vi "GetText.vi"(8 "error in":errorcluster, 11 "channel in":refnum<class "Channel.lvclass">) -> (0 "error out":errorcluster, 1 "additional text":string, 2 "text":string, 3 "channel out":refnum<class "Channel.lvclass">, 4 "glyph":string)   [LabVIEW 2015, in "Channel.lvclass"]
doc: "Copyright 2017 National Instruments Corporation\n\nLicensed under the Apache License, Version 2.0 (the \"License\"); you may not use this file except in compliance with the License. You may obtain a copy of the License at http://www.apache.org/licenses/LICENSE-2.0\nUnless required by applicable law or agreed to in writing, software distributed under the License is distributed on an \"AS IS\" BASIS, WITHOUT WARRANTIES OR CONDITIONS OF ANY KIND, either express or implied. See the License for the specific language governing permissions and limitations under the License."
uses:
  Channel.lvclass
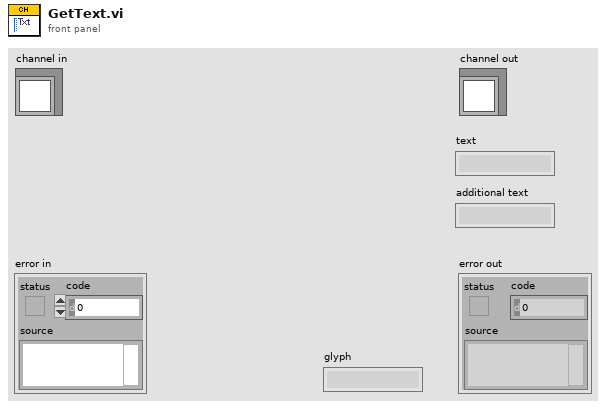
[diagram p1: front panel]
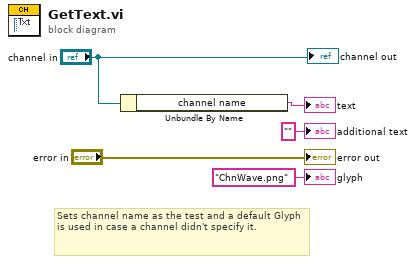
[diagram p0: block diagram]
diagram:
  # "Sets channel name as the test and a default Glyph is used in case a channel didn't specify it."
  n1 = Unbundle By Name("channel in") -> ("channel name"=→"text":string)
  "error out" <- "error in"
  "channel out" <- "channel in"
  "additional text" <- "" ("additional text")
  "glyph" <- "ChnWave.png" ("glyph")
